vi "GetText.vi"(8 "error in":errorcluster, 11 "cRIO in":refnum<class "MainCategoryNode.lvclass">) -> (0 "error out":errorcluster, 1 "additional text":string, 2 "text":string, 3 "cRIO out":refnum<class "MainCategoryNode.lvclass">, 4 "glyph":string)   [LabVIEW 2015, in "MainCategoryNode.lvclass"]
doc: "Copyright 2017 National Instruments Corporation\n\nLicensed under the Apache License, Version 2.0 (the \"License\"); you may not use this file except in compliance with the License. You may obtain a copy of the License at http://www.apache.org/licenses/LICENSE-2.0\nUnless required by applicable law or agreed to in writing, software distributed under the License is distributed on an \"AS IS\" BASIS, WITHOUT WARRANTIES OR CONDITIONS OF ANY KIND, either express or implied. See the License for the specific language governing permissions and limitations under the License."
uses:
  MainCategoryNode.lvclass
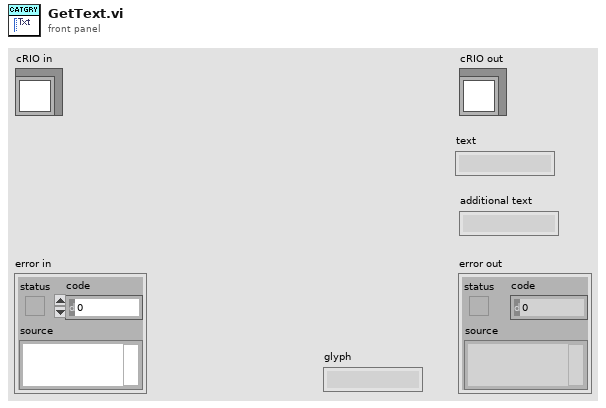
[diagram p1: front panel]
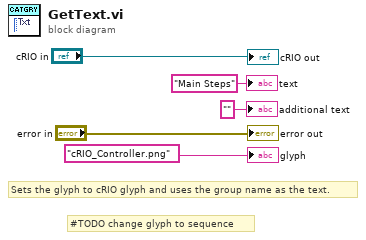
[diagram p0: block diagram]
diagram:
  # "#TODO change glyph to sequence"
  # "Sets the glyph to cRIO glyph and uses the group name as the text."
  "error out" <- "error in"
  "cRIO out" <- "cRIO in"
  "text" <- "Main Steps" ("text")
  "additional text" <- "" ("additional text")
  "glyph" <- "cRIO_Controller.png" ("glyph")
